vi "GetPieceMap.vi"(8 "error in (no error)":errorcluster, 11 "object in":refnum<class "Board.lvclass">) -> (0 "error out":errorcluster, 1 "All Pieces":map{string, i32}[](array[numeric]), 2 "pieceMap":T1, 3 "object out":refnum<class "Board.lvclass">)   [LabVIEW 2020, in "Board.lvclass"]
uses:
  Board.lvclass
  Pieces/typedefs/pieceMap.ctl
  Pieces/Piece.lvclass
  Board.lvclass/Board.ctl
  Pieces/typedefs/pieceType.ctl
  Pieces/Piece.lvclass/Piece.ctl
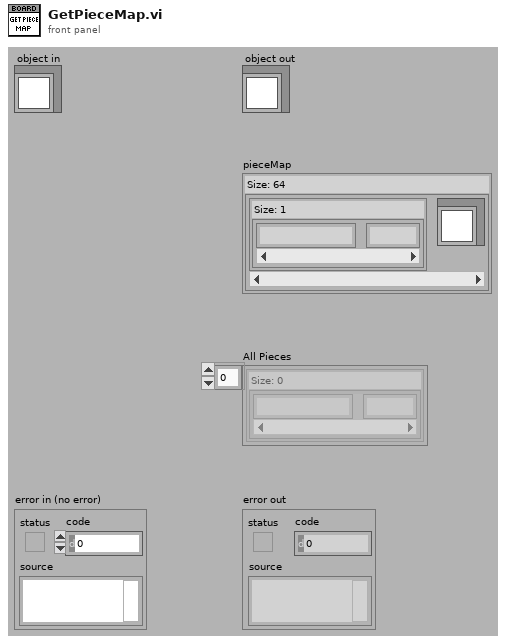
[diagram p1: front panel]
types:
  T1 = typedef "Board.lvclass/pieceMap.ctl" = map{map{string, i32}, refnum<class "Piece.lvclass">}
  T2 = typedef "Piece.lvclass/pieceType.ctl" = enum16{"K", "Q", "R", "N", "B", "P", "none"}
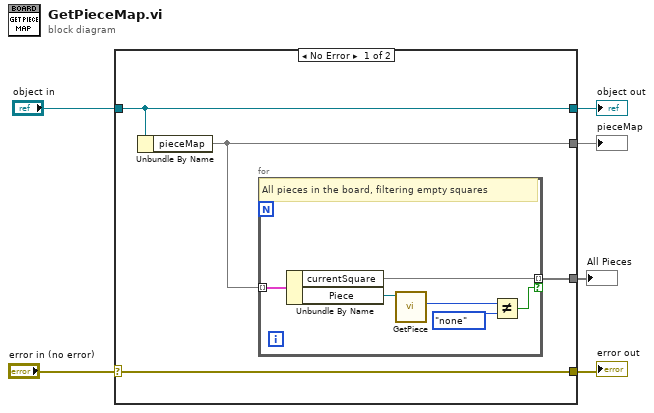
[diagram p0: block diagram]
diagram:
  n1 = case shown="No Error" "error in (no error)" {
    selector: "error in (no error)" -> [w10 w18]
    tunnel: [w10 w18] -> w5
    tunnel: [w9 w17] -> w3
    tunnel: "object in" -> [w9 w17]
    tunnel: [w8 _] -> w2
    tunnel: [w7 _] -> w1
    frame No Error {
      n2 = Unbundle By Name(w9) -> ("pieceMap"=w8:T1)
      n3 = for {
        tunnel: w8 -> [w16] mode=indexing
        tunnel: [w15] -> w7 mode=indexing if=w11
        # "All pieces in the board, filtering empty squares"
        n4 = Unbundle By Name(w16) -> ("currentSquare"=w15:map{string, i32}, "Piece"=w14:refnum<class "Piece.lvclass">)
        n5 = call "GetPiece.vi"("Piece in"=w14) -> ("piece"=w13:T2)  [unwired: 6 in, 4 out]
        n6 = Not Equal?(x=w13, y=pieceType."none") -> (x != y?=w11:bool)
      }
    }
    frame Error {
    }
  }
  "error out" <- w5
  "object out" <- w3
  "pieceMap" <- w2
  "All Pieces" <- w1
